vi "Load Device Signals.vi"(8 "error in":errorcluster, 11 "Config in":refnum<class "Config.lvclass">) -> (0 "error out":errorcluster, 3 "Config out":refnum<class "Config.lvclass">)   [LabVIEW 2023, in "Config.lvlib" / "Config.lvclass"]
uses:
  Config.lvclass
  Config.lvclass/Config.ctl
  builds/Tools/SLL.lvlibp/Methods/Write Device.vi
  builds/Tools/SLL.lvlibp/SLL.lvclass
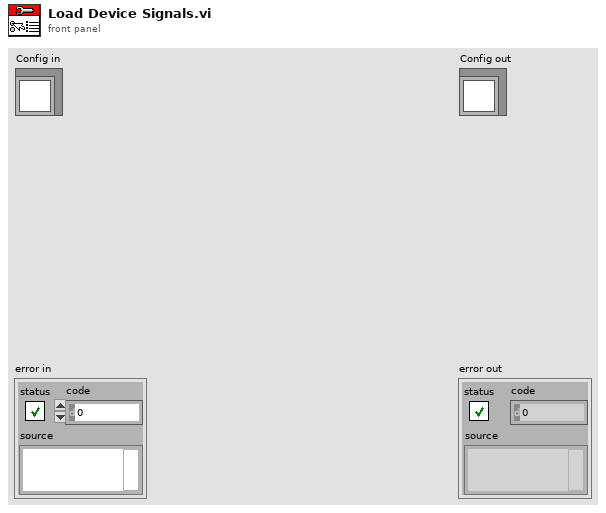
[diagram p1: front panel]
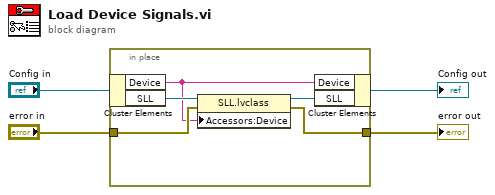
[diagram p0: block diagram]
diagram:
  n1 = in-place {
    in-place-border: "error in" -> [w7]
    in-place-border: [w6] -> w1
    n2 = in-place-cluster #1("Config in") -> ("Device"=w5:string, "SLL"=w9:refnum<class "SLL.lvclass">)
    n3 = property class="SLL.lvclass"(reference=w9, error in=w7, "Accessors:Device"=w5) -> (reference out=w8:refnum<class "SLL.lvclass">, error out=w6:errorcluster)
    n4 = in-place-cluster #1("Device"=w5, "SLL"=w8) -> (→"Config out":refnum<class "Config.lvclass">)
  }
  "error out" <- w1
